vi "Host_ExtendedDetails.vi"() -> ()   [LabVIEW 2018]
doc: "View all sensor readings with a comparison to nominal range."
uses:
  Master/DAQ/Master_DataControl.ctl
  Master/DAQ/TypeDef_cRIOData.ctl
  Master/IMU/TypeDef_IMUData.ctl
  Master/CAN/TypeDef_BMSData.ctl
  Master/CAN/TypeDef_BMS_Status.ctl
  Master/CAN/MotorController/fixedMotorData.ctl
  Master/CAN/MotorController/MotorStatus.ctl
  Globals/Host_DATAALL.vi
  Globals/Host_UDPGLOBALS.vi
panel:
  in  "Motor Enum":T1(ring) caption="Display Motor Data:"
  out "isWarning":bool
  out "targetReached":bool
  out "isVoltEn":bool
  out "isFault":bool
  out "isOperEn":bool
  out "isOn":bool
  out "isReady":bool
  out "Motor Controller State":u16(ring) items=["unknown"=1, "boot-up"=0, "stopped"=4, "operational"=5, "pre-operational"=127, "connection lost"=128]
  out "Motor Alive?":bool
  out "Waveform Graph 3":dbl[](graph)
  in  "Motor Table":string[][](table)
  out "Isolation":bool
  out "BMS Fault":bool
  in  "BMS Enum":T2(ring) caption="Display BMS Data:"
  in  "Close Window":bool
  in  "cRIO Enum":T3(ring) caption="Display Data:"
  out "Waveform Graph 2":dbl[](graph)
  out "Waveform Graph":dbl[](graph)
  out "Min Cell ID":dbl
  out "Max Cell ID":dbl
  out "UDP Display":string caption="UDP Sent"
  in  "BMS Table":string[][](table)
  in  "cRIO IMU Table":string[][](table)
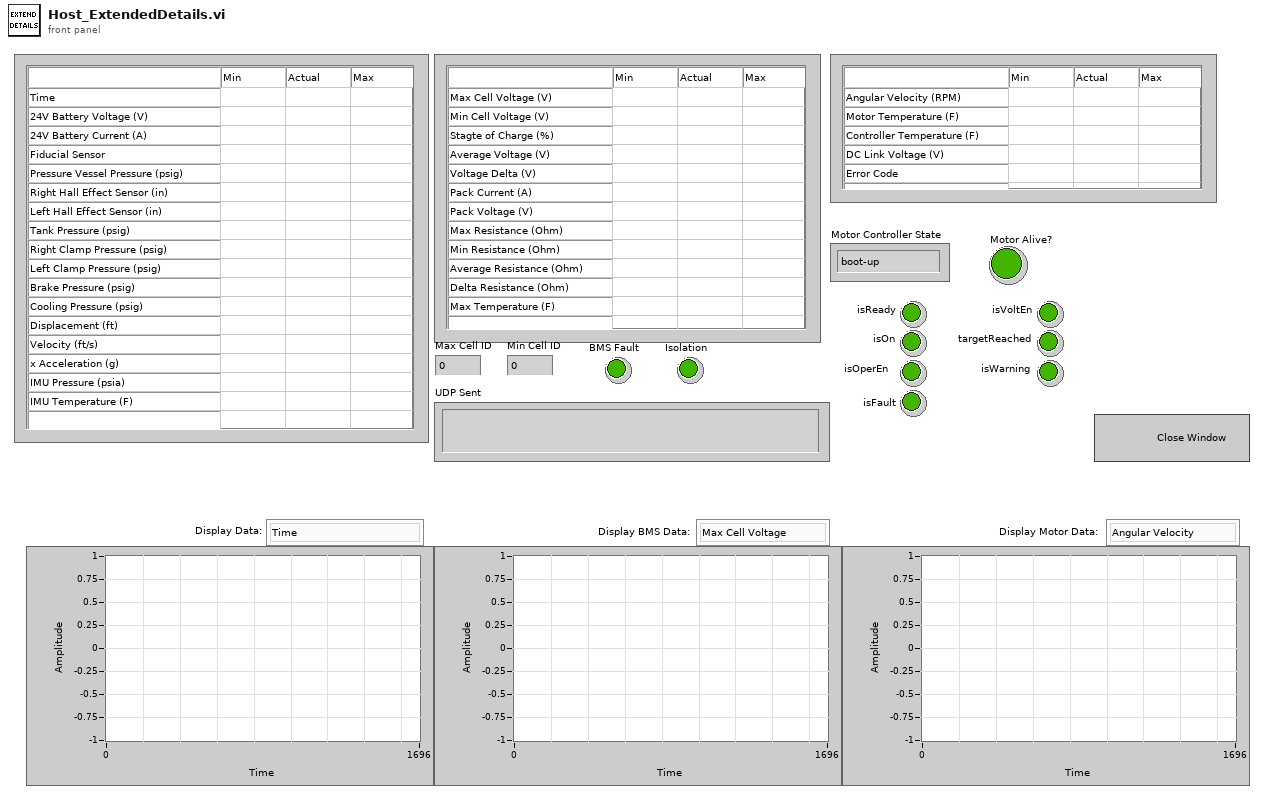
[diagram p1: front panel]
types:
  T1 = enum16{"Angular Velocity", "Motor Temperature", "Controller Temperature", "DC Link Voltage"}
  T2 = enum16{"Max Cell Voltage", "Max Cell ID", "Min Cell Voltage", "Min Cell ID", "State of Charge", "Average Voltage", "Voltage Delta", "Pack Current", "Pack Voltage", "Max Resistance", "Min Resistance", "Average Resistance", "Delta Resistance", "Max Temperature", "Fault", "Isolation"}
  T3 = enum16{"Time", "24V Battery Voltage", "24V Battery Current", "Stripe Count", "Pressure Vessel Pressure", "Flow Sensor", "Fairing Temperature", "Reservoir Temperature", "RIght Hall Effect", "Left Hall Effect", "Tank Pressure", "Right Clamp Pressure", "Left Clamp Pressure", "Brake Pressure", "Cooling Pressure", "DIsplacement", "Velocity", "Acceleration", "Ambient Pressure", "IMU Temperature"}
  T4 = typedef "Master_DataControl.ctl" = cluster{"cRIO Data":T5, "IMU Data":T6, "BMS Data":T7, "Motor Data":T9}
  T5 = typedef "TypeDef_cRIOData.ctl" = cluster{"Time (ms)":dbl, "24V Battery (V)":dbl, "LowV Current (A)":dbl, "Fiducial Sensor (V)":dbl, "PV Pressure (psig)":dbl, "Flow Sensor (V)":dbl, "Temp Fairing (F)":dbl, "Temp Reservoir (F)":dbl, "HallEffect Right (in)":dbl, "HallEffect Left (in)":dbl, "PT Tank (psig)":dbl, "PT Clamp Right (psig)":dbl, "PT Clamp Left (psig)":dbl, "PT Brake (psig)":dbl, "PT Cooling (psig)":dbl, "Displacement (ft)":dbl, "Velocity (ft/s)":dbl}
  T6 = typedef "TypeDef_IMUData.ctl" = cluster{"x acceleration (g)":dbl, "Pressure (psia)":dbl, "Temperature (F)":dbl}
  T7 = typedef "TypeDef_BMSData.ctl" = cluster{"Max Cell Voltage (V)":dbl, "Max Cell ID":dbl, "Min Cell Voltage (V)":dbl, "Min Cell ID":dbl, "State of Charge (%)":dbl, "Average Voltage (V)":dbl, "Voltage Delta (V)":dbl, "Pack Current (A)":dbl, "Pack Voltage (V)":dbl, "Max Resistance (Ohm)":dbl, "Min Resistance (Ohm)":dbl, "Average Resistance (Ohm)":dbl, "Delta Resistance (Ohm)":dbl, "Highest Temperature(F)":dbl, "BmsStatus":T8}
  T8 = typedef "TypeDef_BMS_Status.ctl" = cluster{"isFault":bool, "isolationMonitoring":bool}
  T9 = typedef "fixedMotorData.ctl" = cluster{"Velo (RPM)":dbl, "MotorTemp(F)":dbl, "CtrlTemp(F)":dbl, "DcLinkVolt(V)":dbl, "ErrorCode":dbl, "motorStatus":T10, "isAlive":bool, "motorControllerState":u16}
  T10 = typedef "MotorStatus.ctl" = cluster{"isReady":bool, "isOn":bool, "isOperEn":bool, "isFault":bool, "isVoltEn":bool, "targetReached":bool, "isWarning":bool}
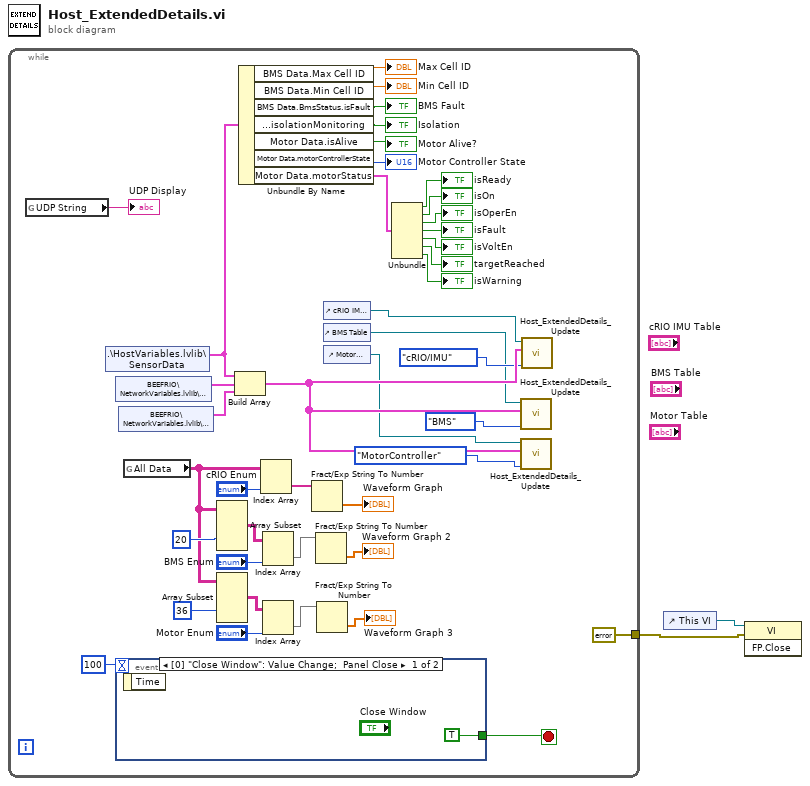
[diagram p0: block diagram]
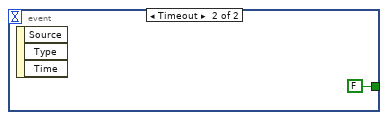
[diagram p2: hidden frame]
diagram:
  n1 = while {
    tunnel: [errorcluster {"status"=FALSE, "code"=0, "source"=""} ("error constant")] -> w1
    stop <- w39 stop-if-true
    n2 = global read "Host_UDPGLOBALS.vi" "UDP String"() -> (→"UDP Display":string)
    n3 = shared-variable ".\\HostVariables.lvlib\\SensorData"() -> (w36:T4)  [unwired: 1 in, 1 out]
    n4 = shared-variable "BEEFRIO\\NetworkVariables.lvlib\\MaxValue"() -> (w44:T4)  [unwired: 1 in, 1 out]
    n5 = event shown="[0] \"Close Window\": Value Change;  Panel Close" {
      selector: _ -> [_ _]
      dyn-events: _ -> [_ _]
      timeout: 100 -> [_ _]
      tunnel: [TRUE FALSE] -> w39
      event "Close Window": Value Change; Panel Close {
        n6 = event-data() -> ()  [unwired: 1 in, 1 out]
      }
      event Timeout {
        n7 = event-data() -> ()  [unwired: 1 in, 3 out]
      }
    }
    n8 = shared-variable "BEEFRIO\\NetworkVariables.lvlib\\MinValue"() -> (w43:T4)  [unwired: 1 in, 1 out]
    n9 = global read "Host_DATAALL.vi" "All Data"() -> (w15:string[][])
    n10 = Array Subset(array=w15, index (col)=20 ("index")) -> (w19:string[][])  [unwired: 3 in]
    n11 = Array Subset(array=w15, index (col)=36 ("index")) -> (w17:string[][])  [unwired: 3 in]
    n12 = Build Array(w36, w44, w43) -> (w9:T4[])
    n13 = Unbundle By Name(w36) -> ("BMS Data.Max Cell ID"=→"Max Cell ID":dbl, "BMS Data.Min Cell ID"=→"Min Cell ID":dbl, "BMS Data.BmsStatus.isFault"=→"BMS Fault":bool, "BMS Data.BmsStatus.isolationMonitoring"=→"Isolation":bool, "Motor Data.isAlive"=→"Motor Alive?":bool, "Motor Data.motorControllerState"=→"Motor Controller State":u16, "Motor Data.motorStatus"=w30:T10)
    n14 = Index Array(array=w15, index (col)="cRIO Enum") -> (element=w13:string[])  [unwired: 1 in]
    n15 = Index Array(array=w19, index (col)="BMS Enum") -> (element=w12:string[])  [unwired: 1 in]
    n16 = Index Array(array=w17, index (col)="Motor Enum") -> (element=w11:string[])  [unwired: 1 in]
    n17 = Fract/Exp String To Number(string=w13) -> (number=→"Waveform Graph":dbl[])  [unwired: 3 in, 1 out]
    n18 = Fract/Exp String To Number(string=w12) -> (number=→"Waveform Graph 2":dbl[])  [unwired: 3 in, 1 out]
    n19 = Fract/Exp String To Number(string=w11) -> (number=→"Waveform Graph 3":dbl[])  [unwired: 3 in, 1 out]
    n20 = control-ref of="cRIO IMU Table"() -> (w3:refnum<vi>)
    n21 = control-ref of="BMS Table"() -> (w4:refnum<vi>)
    n22 = control-ref of="Motor Table"() -> (w5:refnum<vi>)
    n23 = Unbundle(w30) -> ("isReady"=→"isReady":bool, "isOn"=→"isOn":bool, "isOperEn"=→"isOperEn":bool, "isFault"=→"isFault":bool, "isVoltEn"=→"isVoltEn":bool, "targetReached"=→"targetReached":bool, "isWarning"=→"isWarning":bool)
    n24 = call "Host_ExtendedDetails_Update.vi"("reference in"=w4, "Data array in"=w9, "Enum"=enum16{"cRIO/IMU", "BMS", "MotorController"}."BMS") -> ()  [unwired: 8 in]
    n25 = call "Host_ExtendedDetails_Update.vi"("reference in"=w5, "Data array in"=w9, "Enum"=enum16{"cRIO/IMU", "BMS", "MotorController"}."MotorController") -> ()  [unwired: 8 in]
    n26 = call "Host_ExtendedDetails_Update.vi"("reference in"=w3, "Data array in"=w9, "Enum"=enum16{"cRIO/IMU", "BMS", "MotorController"}."cRIO/IMU") -> ()  [unwired: 8 in]
  }
  n27 = control-ref of="This VI"() -> (w2:refnum<vi>)
  n28 = invoke class="VI" method="FP.Close"(reference=w2, error in=w1) -> ()  [unwired: 1 in, 3 out]
